vi "GetSetProgramLoopsLeft.vi"(8 "error in":errorcluster, 9 "Loops left":u16 max=9999 step=1, 10 "get/set":T1=enum."set", 11 "VISA resource name":refnum<visa-resource-name>) -> (0 "error out":errorcluster, 2 "Loops left?":string, 3 "VISA resource name out":refnum<visa-resource-name>)   [LabVIEW 2023, in "Thermotron 8800.lvlib"]
doc: "LLFT\nCommand name: Send or load program loops left\nCommand type: Program status; edit from hold\nDescription: The query command asks the 8800 for the number of loops left to be executed for the current loop. On nested looping, the value is for the inside loop. The 8800 sends an integer to indicate the number of loops left. The edit from hold operation command temporarily changes the current interval’s loop counter.\nSyntax: LLFT? or LLFTn\nWhere n is the number of loops.\nData type: Integer\nQuery example: LLFT?\n8800 response: 8 (There are 8 loops left to be executed for the current loop.)\nOperation example: LLFT15\n8800 response: Changes the loops left counter to 15."
uses:
  Thermotron 8800.lvlib
  Private/get set.ctl
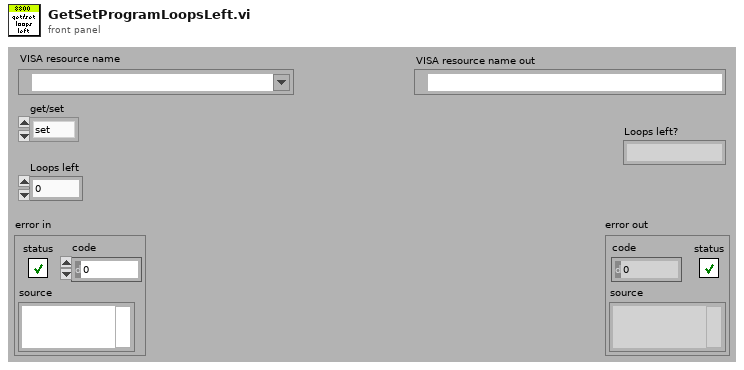
[diagram p1: front panel]
types:
  T1 = typedef "Thermotron 8800.lvlib/get set.ctl" = enum16{"get", "set"}
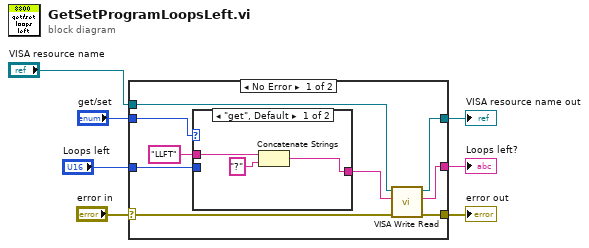
[diagram p0: block diagram]
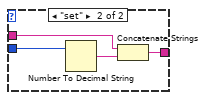
[diagram p2: hidden frame]
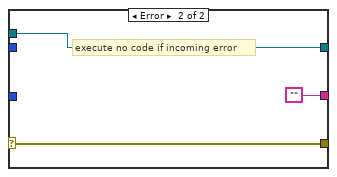
[diagram p3: hidden frame]
diagram:
  n1 = case shown="No Error" "error in" {
    selector: "error in" -> [w8 w25]
    tunnel: "get/set" -> [w16 _]
    tunnel: [w13 ""] -> w3
    tunnel: [w12 w25] -> w6
    tunnel: [w11 w26] -> w4
    tunnel: "VISA resource name" -> [w10 w26]
    tunnel: "Loops left" -> [w9 _]
    frame No Error {
      n2 = case shown="\"get\", Default" w16 {
        tunnel: "LLFT" ("8800 Command") -> [w18 w23]
        tunnel: [w19 w22] -> w14
        tunnel: w9 -> [_ w20]
        frame "get", Default {
          n3 = Concatenate Strings(w18, "?" ("8800 Command")) -> (w19:string)
        }
        frame "set" {
          n4 = Number To Decimal String(number=w20) -> (decimal integer string=w21:string)  [unwired: 1 in]
          n5 = Concatenate Strings(w23, w21) -> (w22:string)
        }
      }
      n6 = call "VISA Write Read.vi"("error in (no error)"=w8, "8800 Command"=w14, "VISA Refnum in"=w10) -> ("error out"=w12:errorcluster, "read buffer"=w13:string, "VISA Refnum out"=w11:refnum<visa-resource-name>)  [unwired: 6 in]
    }
    frame Error {
      # "execute no code if incoming error"
    }
  }
  "VISA resource name out" <- w4
  "error out" <- w6
  "Loops left?" <- w3
